vi "Lifetime at UC Intersection (standard).vi"(8 "Error In":errorcluster, 11 "Data for Pseudo UC Intersections":T1={"Linear Coefficients"={"u"=0.0, "v"=0.0}, "Decay Definition"={"offset: t0"=0.0, "period: T"=0.0, "lifetime: tau"=0.0, "Incident Signal: I"=0.0, "Normalized Decays"=FALSE, "IRF Model"=enum."Dirac", "IRF Parameter 1"=0.0}, "Gates Definitions"={"First Gate: t1"=0.0, "Gate Width: W"=0.0, "Gate Step: d"=0.0, "# Gates: G"=0.0, "Use Gate Center"=FALSE, "Frames/Image: F"=0, "Gates/Frame: L"=0, "Bits/Frame: q"=0, "Multiplicity: p"=0, "Gate Type"=enum."Square", "Gate Edge s"=4.0, "Gate Top Slope"=4.0, "Reversed Sawtooth?"=FALSE, "Computation"=FALSE, "User-defined Gate"={"X Array"=[], "Y Array"=[]}, "Tolerance"=50.0, "Integration"=enum."Item 0", "# Steps"=50.0, "Type of User-defined Function"=enum."Gate"}, "iw"=0.0+0.0i, "Phasor Calculation"=enum."Direct Sum"}) -> (0 "Error Out":errorcluster, 1 "Analytical Solution 1":dbl[unit], 3 "Analytical Solution 2":dbl[unit])   [LabVIEW 2019]
uses:
  Data for Pseudo UC Intersections.ctl
  Decay Definiton.ctl
  IRF Model.ctl
  Gate Definitions.ctl
  Gate Type.ctl
  XY Plot Data.ctl
  Phasor Calculation Type.ctl
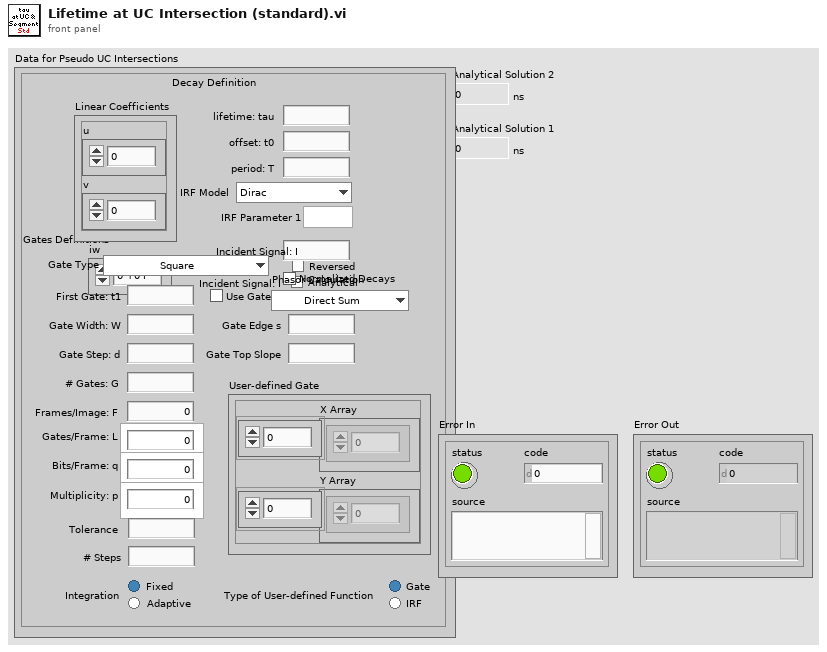
[diagram p1: front panel]
types:
  T1 = typedef "Data for Pseudo UC Intersections.ctl" = cluster{"Linear Coefficients":cluster{"u":dbl, "v":dbl}, "Decay Definition":T2, "Gates Definitions":T4, "iw":cdb, "Phasor Calculation":T7}
  T2 = typedef "Decay Definiton.ctl" = cluster{"offset: t0":ext, "period: T":ext, "lifetime: tau":ext, "Incident Signal: I":ext, "Normalized Decays":bool, "IRF Model":T3, "IRF Parameter 1":ext}
  T3 = typedef "IRF Model.ctl" = enum16{"Dirac", "Exponential"}
  T4 = typedef "Gate Definitions.ctl" = cluster{"First Gate: t1":ext, "Gate Width: W":ext, "Gate Step: d":ext, "# Gates: G":ext, "Use Gate Center":bool, "Frames/Image: F":i32, "Gates/Frame: L":i32, "Bits/Frame: q":i32, "Multiplicity: p":i32, "Gate Type":T5, "Gate Edge s":ext, "Gate Top Slope":ext, "Reversed Sawtooth?":bool, "Computation":bool, "User-defined Gate":T6, "Tolerance":ext, "Integration":enum32{"Item 0", "Item 1"}, "# Steps":ext, "Type of User-defined Function":enum32{"Gate", "IRF"}}
  T5 = typedef "Gate Type.ctl" = enum16{"Square", "Finite Edge Square", "Finite Edge, Tilted Top Square", "Triangle", "Sawtooth", "User-defined"}
  T6 = typedef "XY Plot Data.ctl" = cluster{"X Array":dbl[], "Y Array":dbl[]}
  T7 = typedef "Phasor Calculation Type.ctl" = enum16{"Direct Sum", "Analytical Formula"}
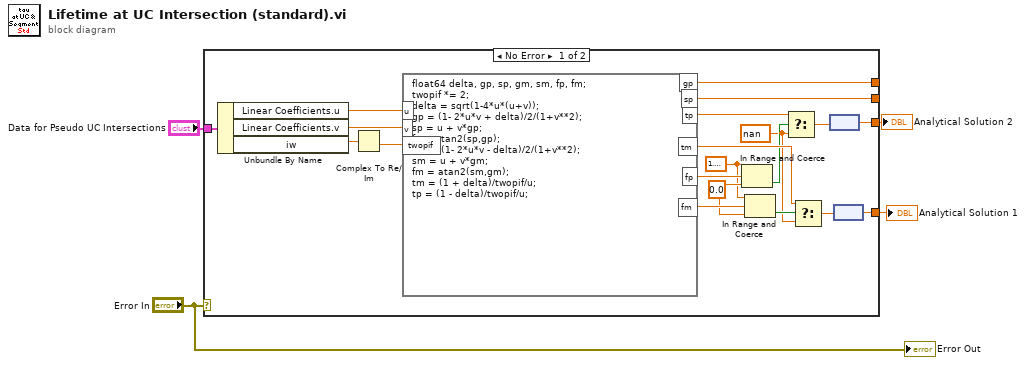
[diagram p0: block diagram]
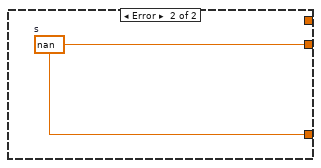
[diagram p2: hidden frame]
diagram:
  n1 = case shown="No Error" "Error In" {
    tunnel: "Data for Pseudo UC Intersections" -> [w24 _]
    tunnel: [w19 w25] -> w3
    tunnel: [w18 w25] -> w2
    tunnel: [w6 _] -> _
    tunnel: [w5 _] -> _
    frame No Error {
      w7 = nan ("f")
      w15 = 0.0 ("lower limit")
      w13 = 1.5707963267948966
      n2 = Unbundle By Name(w24) -> ("Linear Coefficients.u"=w23:dbl, "Linear Coefficients.v"=w22:dbl, "iw"=w21:cdb)
      n3 = Complex To Re/Im(x + iy=w21) -> (y=w20:dbl)  [unwired: 1 out]
      n4 = formula code="float64 delta, gp, sp, gm, sm, fp, fm;\ntwopif *= 2;\ndelta = sqrt(1-4*u*(u+v));\ngp = (1- 2*u*v + delta)/2/(1+v**2);\nsp = u + v*gp;\nfp = atan2(sp,gp);\ngm = (1- 2*u*v - delta)/2/(1+v**2);\nsm = u + v*gm; \nfm = atan2(sm,gm);\ntm = (1 + delta)/twopif/u;\ntp = (1 - delta)/twopif/u;"("u"=w23, "v"=w22, "twopif"=w20) -> ("tp"=w9:dbl, "tm"=w11:dbl, "fp"=w14:dbl, "fm"=w16:dbl, "gp"=w6:dbl, "sp"=w5:dbl)
      n5 = In Range and Coerce(upper limit=w13, x=w14, lower limit=w15) -> (In Range?=w10:bool)  [unwired: 1 out]
      n6 = In Range and Coerce(upper limit=w13, x=w16, lower limit=w15) -> (In Range?=w17:bool)  [unwired: 1 out]
      n7 = Select(t=w9, s=w10, f=w7) -> (s? t:f=w8:dbl)
      n8 = Select(t=w11, s=w17, f=w7) -> (s? t:f=w12:dbl)
      n9 = node(w8) -> (w18:dbl[unit])
      n10 = node(w12) -> (w19:dbl[unit])
    }
    frame Error {
      w25 = dbl[unit] nan  # s
    }
  }
  "Analytical Solution 1" <- w3
  "Analytical Solution 2" <- w2
  "Error Out" <- "Error In"
